vi "Diagnostic.vi"(8 "error in (no error)":errorcluster, 11 "Connection Data In":T1) -> (0 "error out":errorcluster, 3 "Connection Data Out":T1)   [LabVIEW 2014, in "MSX-E3701_dll.lvlib"]
doc: "Encargado de Testear si hay transductores desconectados, si se produjo un corto circuito en alguno de ellos y de rearmarlos."
uses:
  MSX-E3701_dll.lvlib
  Typedef/Connection Data.ctl
  E:/Repositorio Magnis/INF002/v0/Modules/HAL/Drivers/Sync/ADDI-DATA MSX-E3701/API/MX370x.dll
  MX370x.dll
  E:/Repositorio Magnis/INF002/v0/Modules/HAL/Drivers/Sync/ADDI-DATA MSX-E3701/API/MXCommon.dll
  MXCommon.dll
panel:
  out "String":string
  out "Rearm \nTransducers\nStatus":bool
  out "Progress Status":i32(slide) scale=0.0..100.0
  out "Table":string[][](table)=[["-", "-"], ["-", "-"], ["-", "-"], ["-", "-"], ["-", "-"], ["-", "-"], ["-", "-"], ["-", "-"], ["-", "-"], ["-", "-"], ["-", "-"], ["-", "-"], ["-", "-"], ["-", "-"], ["-", "-"], ["-", "-"], ["-", "-"]]
  in  "Rearm Transducers":bool
  in  "ConnectionStatus":bool
  in  "ShortCircuit":bool
  in  "Start":bool
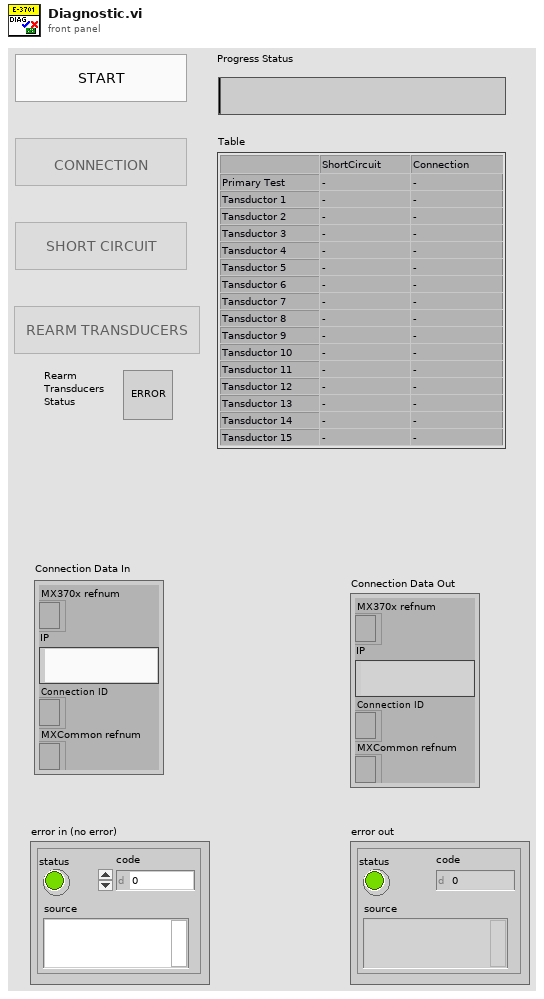
[diagram p1: front panel]
types:
  T1 = typedef "MSX-E3701_dll.lvlib/Connection Data.ctl" = cluster{"MX370x refnum":refnum<k24>, "IP":string, "Connection ID ":refnum<k5>, "MXCommon refnum":refnum<k24>}
  T2 = enum8{"Enabled", "Disabled", "Disabled and Grayed Out"}
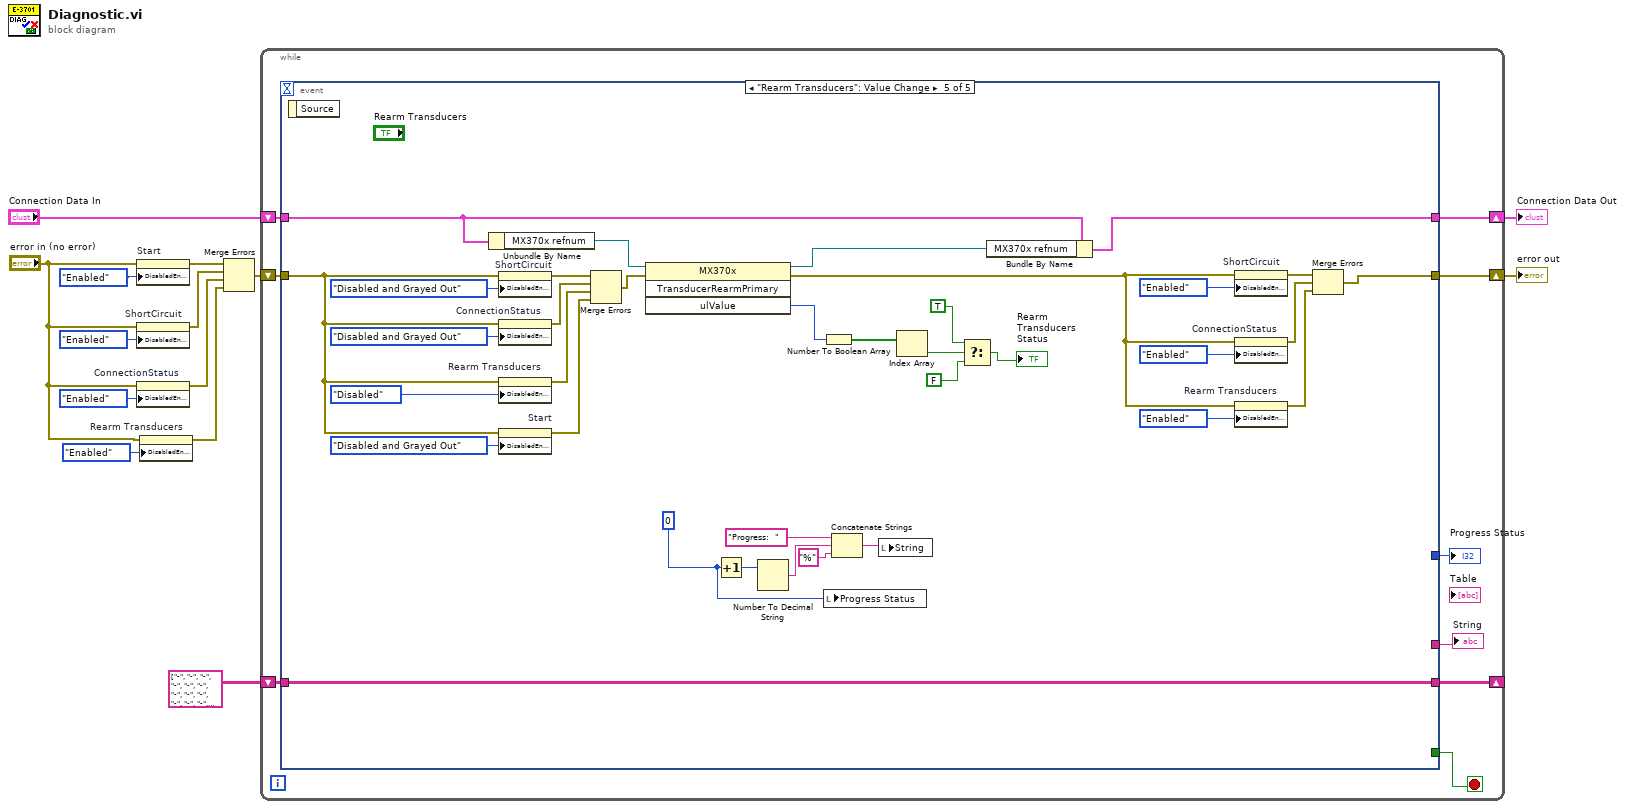
[diagram p0: block diagram]
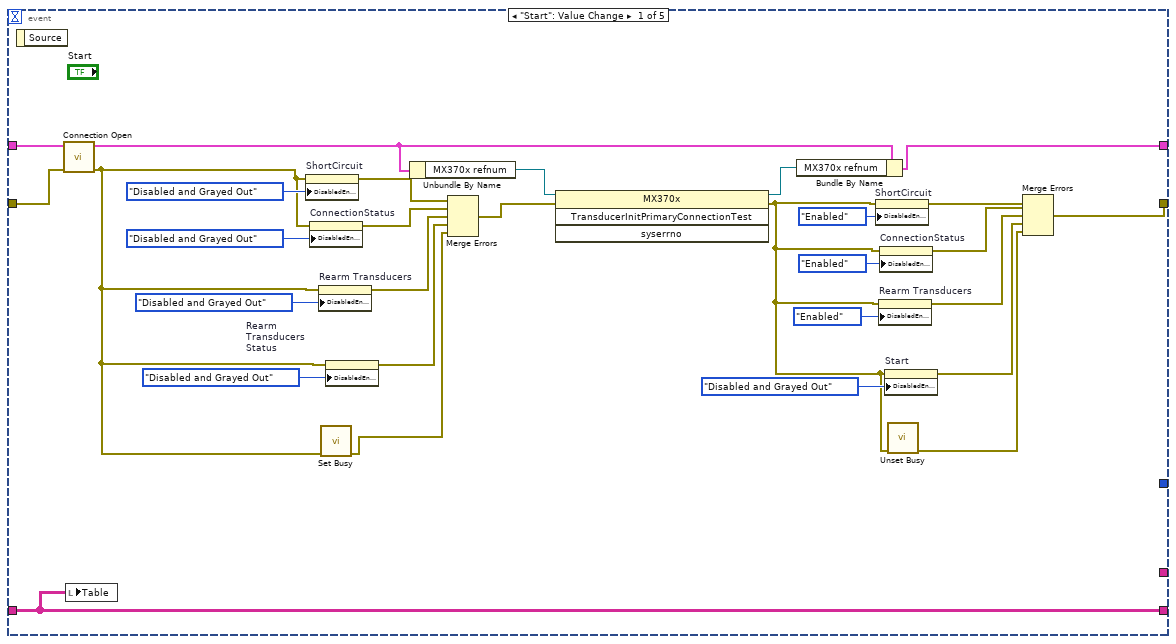
[diagram p2: hidden frame]
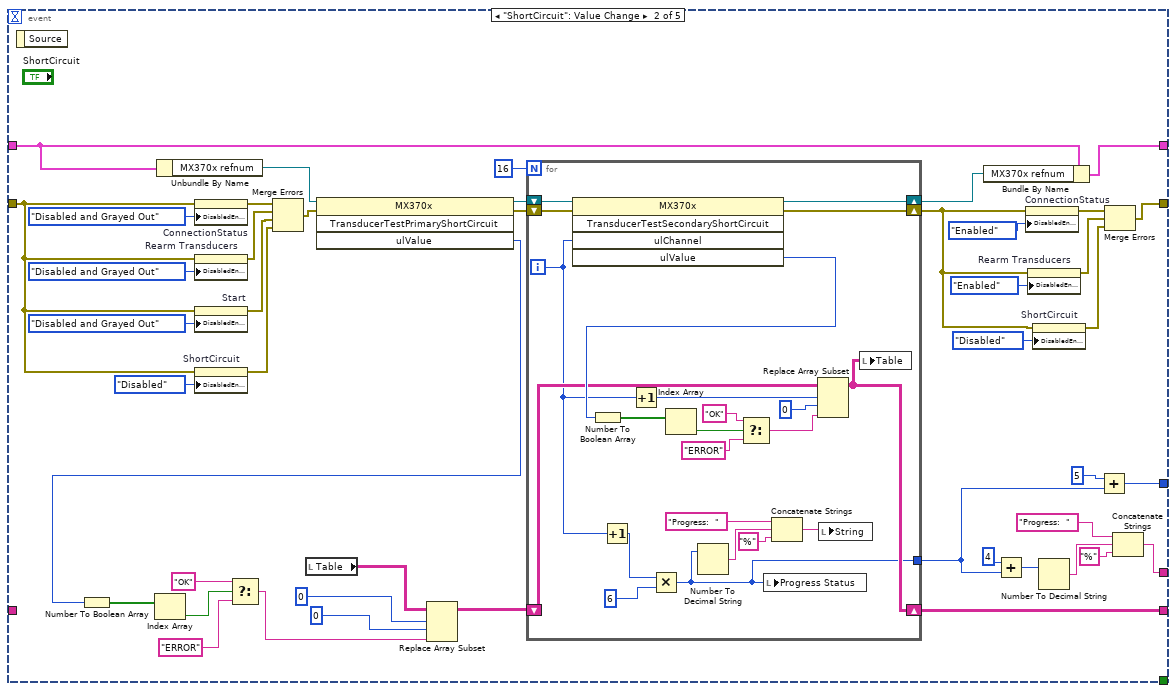
[diagram p3: hidden frame]
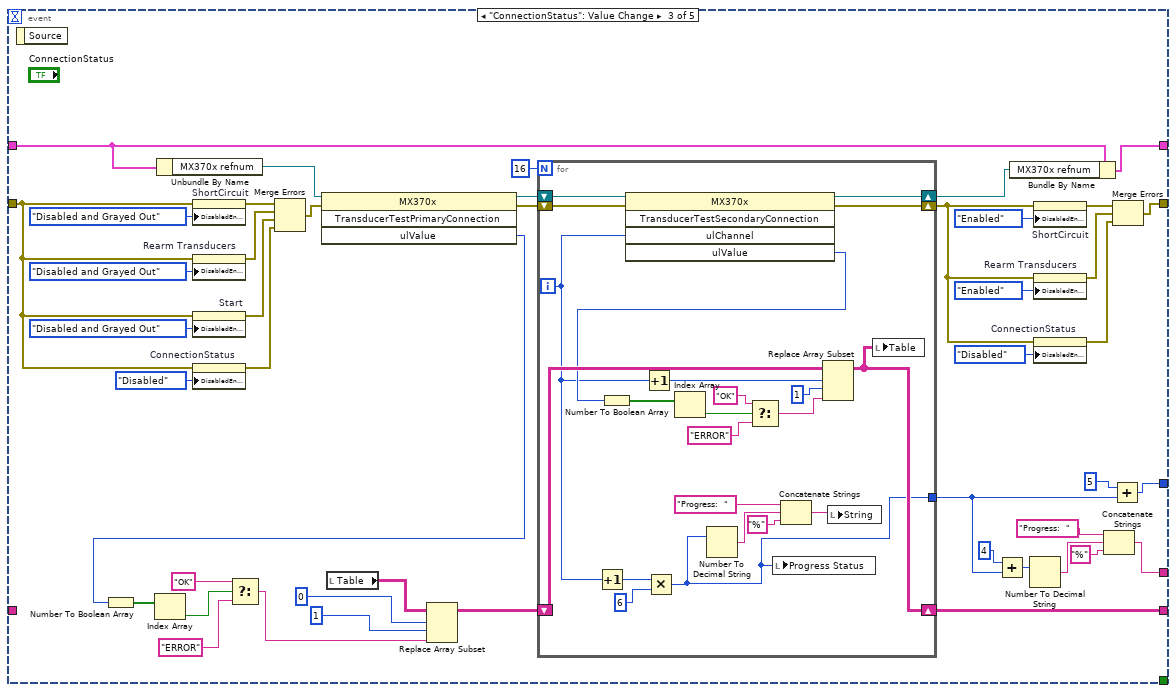
[diagram p4: hidden frame]
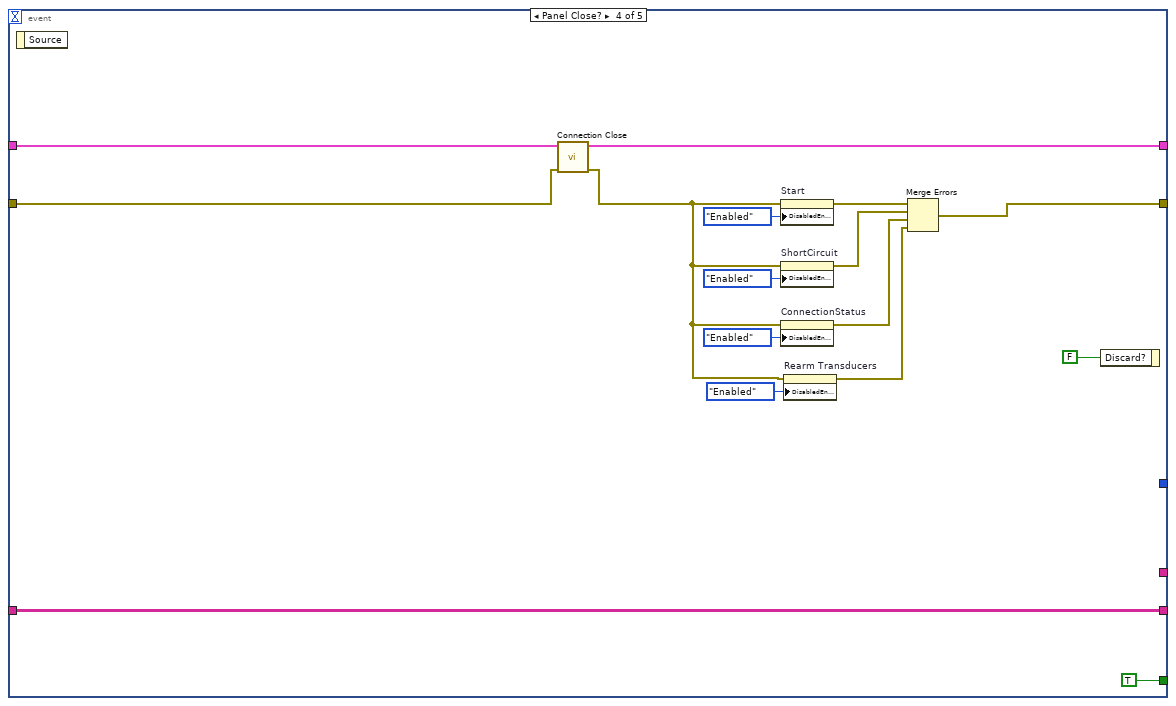
[diagram p5: hidden frame]
diagram:
  n1 = property on="Start" class="Bool"(error in="error in (no error)", "DisabledEnum"=T2."Enabled" ("Disabled")) -> (error out=w6:errorcluster)  [unwired: 1 in, 1 out]
  n2 = property on="ShortCircuit" class="Bool"(error in="error in (no error)", "DisabledEnum"=T2."Enabled" ("Disabled")) -> (error out=w7:errorcluster)  [unwired: 1 in, 1 out]
  n3 = property on="ConnectionStatus" class="Bool"(error in="error in (no error)", "DisabledEnum"=T2."Enabled" ("Disabled")) -> (error out=w8:errorcluster)  [unwired: 1 in, 1 out]
  n4 = property on="Rearm Transducers" class="Bool"(error in="error in (no error)", "DisabledEnum"=T2."Enabled" ("Disabled")) -> (error out=w10:errorcluster)  [unwired: 1 in, 1 out]
  n5 = Merge Errors(w6, w7, w8, w10) -> (w1:errorcluster)
  n6 = while {
    shift-right: [w22] -> w13
    shift-left: "Connection Data In" -> [w21]
    shift-right: [w19] -> w12
    shift-left: w1 -> [w20]
    shift-right: [w17] -> _
    shift-left: string[][] [["-", "-"], ["-", "-"], ["-", "-"], ["-", "-"], ["-", "-"], ["-", "-"], ["-", "-"], ["-", "-"], ["-", "-"], ["-", "-"], ["-", "-"], ["-", "-"], ["-", "-"], ["-", "-"], ["-", "-"], ["-", "-"], ["-", "-"]] ("Table") -> [w18]
    stop <- w23 stop-if-true
    n7 = event shown="[4] \"Rearm Transducers\": Value Change" {
      selector: _ -> [_ _ _ _ _]
      dyn-events: _ -> [_ _ _ _ _]
      timeout: _ -> [_ _ _ _ _]
      tunnel: [_ _ _ TRUE ("Close") _] -> w23
      tunnel: [w51 w70 w161 w198 w234] -> w22
      tunnel: w21 -> [w49 w81 w162 w199 w235]
      tunnel: [w38 w71 w136 w190 w223] -> w19
      tunnel: w20 -> [w47 w56 w124 w197 w206]
      tunnel: w18 -> [w37 _ _ w202 w233]
      tunnel: [_ w62 w155 _ _] -> w15
      tunnel: [w37 w82 w143 w202 w233] -> w17
      tunnel: [_ w63 w131 _ _] -> w16
      event "Start": Value Change {
        n8 = event-data() -> ()  [unwired: 1 in, 1 out]
        n9 = call "Connection Open.vi"("Error In"=w47, "Connection Data In"=w49) -> ("Error Out"=w27:errorcluster, "Connection Data Out"=w48:T1)  [unwired: 8 in]
        n10 = local write "Table"(w37) -> ()
        n11 = property on="ShortCircuit" class="Bool"(error in=w27, "DisabledEnum"=T2."Disabled and Grayed Out" ("Disabled")) -> (error out=w46:errorcluster)  [unwired: 1 in, 1 out]
        n12 = property on="ConnectionStatus" class="Bool"(error in=w27, "DisabledEnum"=T2."Disabled and Grayed Out" ("Disabled")) -> (error out=w35:errorcluster)  [unwired: 1 in, 1 out]
        n13 = property on="Rearm Transducers" class="Bool"(error in=w27, "DisabledEnum"=T2."Disabled and Grayed Out" ("Disabled")) -> (error out=w34:errorcluster)  [unwired: 1 in, 1 out]
        n14 = call <vilib>:"Set Busy.vi"("error in (no error)"=w27) -> ("error out"=w26:errorcluster)  [unwired: 9 in, 1 out]
        n15 = property on="Rearm \nTransducers\nStatus" class="Bool (strict)"(error in=w27, "DisabledEnum"=T2."Disabled and Grayed Out" ("Disabled")) -> (error out=w28:errorcluster)  [unwired: 1 in, 1 out]
        n16 = Unbundle By Name(w48) -> ("MX370x refnum"=w52:refnum<k24>)
        n17 = Merge Errors(w46, w35, w34, w28, w26) -> (w43:errorcluster)
        n18 = invoke class="MX370x" method="TransducerInitPrimaryConnectionTest"(reference=w52, error in=w43) -> (reference out=w50:refnum<k24>, error out=w25:errorcluster)  [unwired: 2 in, 2 out]
        n19 = Bundle By Name(cluster=w48, "MX370x refnum"=w50) -> (w51:T1)
        n20 = property on="ShortCircuit" class="Bool"(error in=w25, "DisabledEnum"=T2."Enabled" ("Disabled")) -> (error out=w39:errorcluster)  [unwired: 1 in, 1 out]
        n21 = property on="Rearm Transducers" class="Bool"(error in=w25, "DisabledEnum"=T2."Enabled" ("Disabled")) -> (error out=w32:errorcluster)  [unwired: 1 in, 1 out]
        n22 = property on="ConnectionStatus" class="Bool"(error in=w25, "DisabledEnum"=T2."Enabled" ("Disabled")) -> (error out=w42:errorcluster)  [unwired: 1 in, 1 out]
        n23 = property on="Start" class="Bool"(error in=w25, "DisabledEnum"=T2."Disabled and Grayed Out" ("Disabled")) -> (error out=w30:errorcluster)  [unwired: 1 in, 1 out]
        n24 = call <vilib>:"Unset Busy.vi"("error in (no error)"=w25) -> ("error out"=w24:errorcluster)  [unwired: 10 in]
        n25 = Merge Errors(w39, w42, w32, w30, w24) -> (w38:errorcluster)
      }
      event "ShortCircuit": Value Change {
        n26 = event-data() -> ()  [unwired: 1 in, 1 out]
        n27 = Unbundle By Name(w81) -> ("MX370x refnum"=w91:refnum<k24>)
        n28 = property on="ConnectionStatus" class="Bool"(error in=w56, "DisabledEnum"=T2."Disabled and Grayed Out" ("Disabled")) -> (error out=w78:errorcluster)  [unwired: 1 in, 1 out]
        n29 = property on="Rearm Transducers" class="Bool"(error in=w56, "DisabledEnum"=T2."Disabled and Grayed Out" ("Disabled")) -> (error out=w77:errorcluster)  [unwired: 1 in, 1 out]
        n30 = property on="Start" class="Bool"(error in=w56, "DisabledEnum"=T2."Disabled and Grayed Out" ("Disabled")) -> (error out=w58:errorcluster)  [unwired: 1 in, 1 out]
        n31 = property on="ShortCircuit" class="Bool"(error in=w56, "DisabledEnum"=T2."Disabled" ("Disabled")) -> (error out=w57:errorcluster)  [unwired: 1 in, 1 out]
        n32 = Merge Errors(w78, w77, w58, w57) -> (w76:errorcluster)
        n33 = local read "Table"() -> (w87:string[][])
        n34 = invoke class="MX370x" method="TransducerTestPrimaryShortCircuit"(reference=w91, error in=w76) -> (reference out=w88:refnum<k24>, error out=w89:errorcluster, "ulValue"=w97:u64)  [unwired: 2 in, 1 out]
        n35 = Number To Boolean Array(number=w97) -> (Boolean array=w96:bool[])
        n36 = Index Array(array=w96) -> (element=w95:bool)  [unwired: 1 in]
        n37 = Select(t="OK" ("String"), s=w95, f="ERROR" ("String")) -> (s? t:f=w84:string)
        n38 = Replace Array Subset(array=w87, new element=w84, index (row)=0, index (col)=0 ("disabled index (col)")) -> (w83:string[][])
        n39 = for {
          N: 16 -> [_]
          shift-right: [w116] -> w90
          shift-left: w88 -> [w119]
          shift-right: [w117] -> w54
          shift-left: w89 -> [w118]
          shift-right: [w102] -> w82
          shift-left: w83 -> [w103]
          tunnel: [w98] -> w61
          i -> [w99]
          n40 = invoke class="MX370x" method="TransducerTestSecondaryShortCircuit"(reference=w119, error in=w118, "ulChannel"=w99) -> (reference out=w116:refnum<k24>, error out=w117:errorcluster, "ulValue"=w107:u64)  [unwired: 2 in, 2 out]
          n41 = Number To Boolean Array(number=w107) -> (Boolean array=w115:bool[])
          n42 = Increment(x=w99) -> (x+1=w101:i32)
          n43 = Increment(x=w99) -> (x+1=w106:i32)
          n44 = Multiply(x=w101, y=6) -> (x*y=w98:i32)
          n45 = Index Array(array=w115) -> (element=w114:bool)  [unwired: 1 in]
          n46 = Number To Decimal String(number=w98) -> (decimal integer string=w109:string)  [unwired: 1 out]
          n47 = Select(t="OK" ("String"), s=w114, f="ERROR" ("String")) -> (s? t:f=w104:string)
          n48 = local write "Progress Status"(w98) -> ()
          n49 = Concatenate Strings("Progress:  ", w109, "%") -> (w111:string)
          n50 = Replace Array Subset(array=w103, new element=w104, index (row)=w106, index (col)=0) -> (w102:string[][])
          n51 = local write "String"(w111) -> ()
          n52 = local write "Table"(w102) -> ()
        }
        n53 = Bundle By Name(cluster=w81, "MX370x refnum"=w90) -> (w70:T1)
        n54 = Add(x=4, y=w61) -> (x+y=w64:i32)
        n55 = property on="ConnectionStatus" class="Bool"(error in=w54, "DisabledEnum"=T2."Enabled" ("Disabled")) -> (error out=w72:errorcluster)  [unwired: 1 in, 1 out]
        n56 = property on="Rearm Transducers" class="Bool"(error in=w54, "DisabledEnum"=T2."Enabled" ("Disabled")) -> (error out=w73:errorcluster)  [unwired: 1 in, 1 out]
        n57 = property on="ShortCircuit" class="Bool"(error in=w54, "DisabledEnum"=T2."Disabled" ("Disabled")) -> (error out=w53:errorcluster)  [unwired: 1 in, 1 out]
        n58 = Number To Decimal String(number=w64) -> (decimal integer string=w67:string)  [unwired: 1 out]
        n59 = Add(x=5, y=w61) -> (x+y=w62:i32)
        n60 = Merge Errors(w72, w73, w53) -> (w71:errorcluster)
        n61 = Concatenate Strings("Progress:  ", w67, "%") -> (w63:string)
      }
      event "ConnectionStatus": Value Change {
        n62 = event-data() -> ()  [unwired: 1 in, 1 out]
        n63 = Unbundle By Name(w162) -> ("MX370x refnum"=w160:refnum<k24>)
        n64 = property on="ShortCircuit" class="Bool"(error in=w124, "DisabledEnum"=T2."Disabled and Grayed Out" ("Disabled")) -> (error out=w141:errorcluster)  [unwired: 1 in, 1 out]
        n65 = property on="Rearm Transducers" class="Bool"(error in=w124, "DisabledEnum"=T2."Disabled and Grayed Out" ("Disabled")) -> (error out=w140:errorcluster)  [unwired: 1 in, 1 out]
        n66 = property on="Start" class="Bool"(error in=w124, "DisabledEnum"=T2."Disabled and Grayed Out" ("Disabled")) -> (error out=w125:errorcluster)  [unwired: 1 in, 1 out]
        n67 = property on="ConnectionStatus" class="Bool"(error in=w124, "DisabledEnum"=T2."Disabled" ("Disabled")) -> (error out=w123:errorcluster)  [unwired: 1 in, 1 out]
        n68 = Merge Errors(w141, w140, w125, w123) -> (w139:errorcluster)
        n69 = invoke class="MX370x" method="TransducerTestPrimaryConnection"(reference=w160, error in=w139) -> (reference out=w159:refnum<k24>, error out=w164:errorcluster, "ulValue"=w144:u64)  [unwired: 2 in, 1 out]
        n70 = Number To Boolean Array(number=w144) -> (Boolean array=w146:bool[])
        n71 = Index Array(array=w146) -> (element=w147:bool)  [unwired: 1 in]
        n72 = Select(t="OK" ("String"), s=w147, f="ERROR" ("String")) -> (s? t:f=w153:string)
        n73 = local read "Table"() -> (w150:string[][])
        n74 = Replace Array Subset(array=w150, new element=w153, index (row)=0, index (col)=1 ("disabled index (col)")) -> (w145:string[][])
        n75 = for {
          N: 16 -> [_]
          shift-right: [w186] -> w120
          shift-left: w164 -> [w185]
          shift-right: [w184] -> w163
          shift-left: w159 -> [w183]
          shift-right: [w169] -> w143
          shift-left: w145 -> [w171]
          tunnel: [w165] -> w129
          i -> [w168]
          n76 = Increment(x=w168) -> (x+1=w167:i32)
          n77 = invoke class="MX370x" method="TransducerTestSecondaryConnection"(reference=w183, error in=w185, "ulChannel"=w168) -> (reference out=w184:refnum<k24>, error out=w186:errorcluster, "ulValue"=w170:u64)  [unwired: 2 in, 2 out]
          n78 = Number To Boolean Array(number=w170) -> (Boolean array=w172:bool[])
          n79 = Increment(x=w168) -> (x+1=w180:i32)
          n80 = Multiply(x=w167, y=6) -> (x*y=w165:i32)
          n81 = Index Array(array=w172) -> (element=w173:bool)  [unwired: 1 in]
          n82 = Number To Decimal String(number=w165) -> (decimal integer string=w178:string)  [unwired: 1 out]
          n83 = Select(t="OK" ("String"), s=w173, f="ERROR" ("String")) -> (s? t:f=w182:string)
          n84 = local write "Progress Status"(w165) -> ()
          n85 = Concatenate Strings("Progress:  ", w178, "%") -> (w176:string)
          n86 = Replace Array Subset(array=w171, new element=w182, index (row)=w180, index (col)=1) -> (w169:string[][])
          n87 = local write "String"(w176) -> ()
          n88 = local write "Table"(w169) -> ()
        }
        n89 = Add(x=4, y=w129) -> (x+y=w128:i32)
        n90 = Bundle By Name(cluster=w162, "MX370x refnum"=w163) -> (w161:T1)
        n91 = Number To Decimal String(number=w128) -> (decimal integer string=w133:string)  [unwired: 1 out]
        n92 = property on="ShortCircuit" class="Bool"(error in=w120, "DisabledEnum"=T2."Enabled" ("Disabled")) -> (error out=w135:errorcluster)  [unwired: 1 in, 1 out]
        n93 = property on="Rearm Transducers" class="Bool"(error in=w120, "DisabledEnum"=T2."Enabled" ("Disabled")) -> (error out=w137:errorcluster)  [unwired: 1 in, 1 out]
        n94 = property on="ConnectionStatus" class="Bool"(error in=w120, "DisabledEnum"=T2."Disabled" ("Disabled")) -> (error out=w121:errorcluster)  [unwired: 1 in, 1 out]
        n95 = Concatenate Strings("Progress:  ", w133, "%") -> (w131:string)
        n96 = Add(x=5, y=w129) -> (x+y=w155:i32)
        n97 = Merge Errors(w135, w137, w121) -> (w136:errorcluster)
      }
      event Panel Close? {
        n98 = event-data() -> ()  [unwired: 1 in, 1 out]
        n99 = call "Connection Close.vi"("error in (no error)"=w197, "Connection Data In"=w199) -> ("error out"=w187:errorcluster, "Connection Data Out"=w198:T1)  [unwired: 8 in]
        n100 = property on="Start" class="Bool"(error in=w187, "DisabledEnum"=T2."Enabled" ("Disabled")) -> (error out=w193:errorcluster)  [unwired: 1 in, 1 out]
        n101 = property on="ShortCircuit" class="Bool"(error in=w187, "DisabledEnum"=T2."Enabled" ("Disabled")) -> (error out=w192:errorcluster)  [unwired: 1 in, 1 out]
        n102 = property on="ConnectionStatus" class="Bool"(error in=w187, "DisabledEnum"=T2."Enabled" ("Disabled")) -> (error out=w191:errorcluster)  [unwired: 1 in, 1 out]
        n103 = property on="Rearm Transducers" class="Bool"(error in=w187, "DisabledEnum"=T2."Enabled" ("Disabled")) -> (error out=w188:errorcluster)  [unwired: 1 in, 1 out]
        n104 = Merge Errors(w193, w192, w191, w188) -> (w190:errorcluster)
        n105 = event-data("Discard?"=FALSE) -> ()  [unwired: 1 in, 1 out]
      }
      event "Rearm Transducers": Value Change {
        w214 = 0
        n106 = event-data() -> ()  [unwired: 1 in, 1 out]
        n107 = Unbundle By Name(w235) -> ("MX370x refnum"=w237:refnum<k24>)
        n108 = property on="ShortCircuit" class="Bool"(error in=w206, "DisabledEnum"=T2."Disabled and Grayed Out" ("Disabled")) -> (error out=w220:errorcluster)  [unwired: 1 in, 1 out]
        n109 = property on="ConnectionStatus" class="Bool"(error in=w206, "DisabledEnum"=T2."Disabled and Grayed Out" ("Disabled")) -> (error out=w219:errorcluster)  [unwired: 1 in, 1 out]
        n110 = property on="Rearm Transducers" class="Bool"(error in=w206, "DisabledEnum"=T2."Disabled" ("Disabled")) -> (error out=w209:errorcluster)  [unwired: 1 in, 1 out]
        n111 = property on="Start" class="Bool"(error in=w206, "DisabledEnum"=T2."Disabled and Grayed Out" ("Disabled")) -> (error out=w207:errorcluster)  [unwired: 1 in, 1 out]
        n112 = Merge Errors(w220, w219, w209, w207) -> (w216:errorcluster)
        n113 = invoke class="MX370x" method="TransducerRearmPrimary"(reference=w237, error in=w216) -> (reference out=w236:refnum<k24>, error out=w203:errorcluster, "ulValue"=w230:u64)  [unwired: 2 in, 1 out]
        n114 = Increment(x=w214) -> (x+1=w215:i32)
        n115 = Number To Decimal String(number=w215) -> (decimal integer string=w228:string)  [unwired: 1 out]
        n116 = Number To Boolean Array(number=w230) -> (Boolean array=w232:bool[])
        n117 = local write "Progress Status"(w214) -> ()
        n118 = Concatenate Strings("Progress:  ", w228, "%") -> (w226:string)
        n119 = local write "String"(w226) -> ()
        n120 = Index Array(array=w232) -> (element=w231:bool)  [unwired: 1 in]
        n121 = Select(t=TRUE, s=w231, f=FALSE) -> (s? t:f=→"Rearm \nTransducers\nStatus":bool)
        n122 = Bundle By Name(cluster=w235, "MX370x refnum"=w236) -> (w234:T1)
        n123 = property on="ShortCircuit" class="Bool"(error in=w203, "DisabledEnum"=T2."Enabled" ("Disabled")) -> (error out=w225:errorcluster)  [unwired: 1 in, 1 out]
        n124 = property on="ConnectionStatus" class="Bool"(error in=w203, "DisabledEnum"=T2."Enabled" ("Disabled")) -> (error out=w224:errorcluster)  [unwired: 1 in, 1 out]
        n125 = property on="Rearm Transducers" class="Bool"(error in=w203, "DisabledEnum"=T2."Enabled" ("Disabled")) -> (error out=w204:errorcluster)  [unwired: 1 in, 1 out]
        n126 = Merge Errors(w225, w224, w204) -> (w223:errorcluster)
      }
    }
    "String" <- w16
    "Progress Status" <- w15
  }
  "error out" <- w12
  "Connection Data Out" <- w13
